vi "Autonomous Independent.vi"() -> ()   [LabVIEW 2016]
doc: "This VI is called when autonomous begins, and will automatically be terminated when autonomous ends. You can carry out timed or sensor driven robot movement independently without needing to return to the caller."
uses:
  <vilib>/Rock Robotics/WPI/Utilities/WPI_GetSetVariantRefNum.vi
  <vilib>/Rock Robotics/Network Tables/NT Read String.vi
  <vilib>/Rock Robotics/Network Tables/NT Write Numeric Array.vi
  <vilib>/Rock Robotics/WPI/RobotDrive/WPI_RobotDriveArcadeDrive_Standard(NoSaturation).vi
panel:
  out "Current Movement, for debugging":T1 {"Y Joystick Value" scale=1.0..-1.0; "X Joystick Value" scale=-1.0..1.0}
  in  "Array of robot movements":T2(array[cluster])=[{"X Joystick Value"=0.39393939393939403, "Y Joystick Value"=0.0, "Delay (sec)"=1.0, "Movement Name"="turn"}, {"X Joystick Value"=-0.3737373737373737, "Y Joystick Value"=0.0, "Delay (sec)"=1.0, "Movement Name"="turn back"}] {"Y Joystick Value" scale=1.0..-1.0; "X Joystick Value" scale=-1.0..1.0}
  # "Be sure to right-click and choose Data Operations>>Make Current Value default if you want to save the array values with the VI"
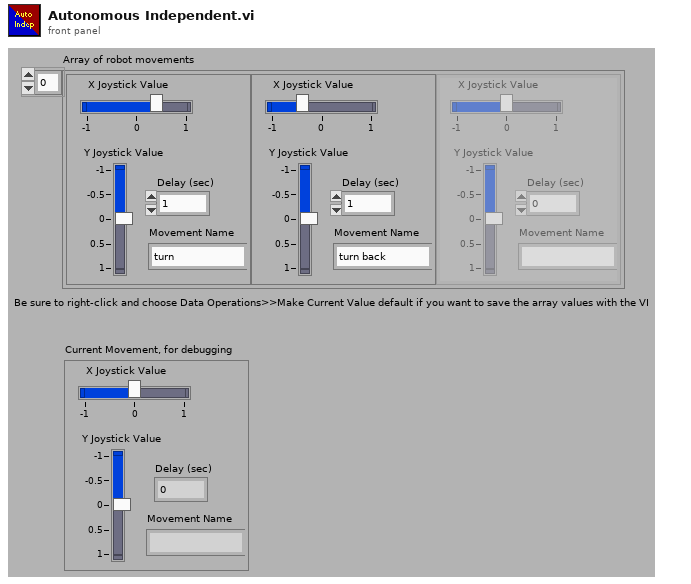
[diagram p1: front panel]
types:
  T1 = cluster{"X Joystick Value":dbl, "Y Joystick Value":dbl, "Delay (sec)":dbl, "Movement Name":string}
  T2 = cluster{"X Joystick Value":dbl, "Y Joystick Value":dbl, "Delay (sec)":dbl, "Movement Name":string}[]
  T3 = typedef "WPI_JoystickDevRef.ctl" = cluster{"Device":T4}
  T4 = typedef "WPI_JoystickDeviceEnum.ctl" = enum16{"USB 0", "USB 1", "USB 2", "USB 3", "USB 4", "USB 5"}
  T5 = typedef "WPI_RobotDriveDevRef.ctl" = cluster{"DevStatus":errorcluster, "Motors[]":T6[], "Square Inputs":bool, "Max Output":dbl}
  T6 = typedef "WPI_MotorControlDeviceRef.ctl" = cluster{"DeviceStatus":errorcluster, "Type":T7, "PWM":cluster{"PWM Channel":T8, "DeadBand":T9}, "CAN":cluster{"Device Number":u8, "SetOutput VI Ref":variant, "GetOutput VI Ref":variant, "Enable VI Ref":variant, "Disable VI Ref":variant, "Data":variant}, "Invert":bool}
  T7 = typedef "WPI_MotorControlType.ctl" = enum16{"PWM", "CAN"}
  T8 = typedef "FPGA_DIOPWMChannel.ctl" = enum8{"PWM 0", "PWM 1", "PWM 2", "PWM 3", "PWM 4", "PWM 5", "PWM 6", "PWM 7", "PWM 8", "PWM 9", "PWM MXP 0", "PWM MXP 1", "PWM MXP 2", "PWM MXP 3", "PWM MXP 4", "PWM MXP 5", "PWM MXP 6", "PWM MXP 7", "PWM MXP 8", "PWM MXP 9", "Invalid"}
  T9 = typedef "WPI_PWMDeadband.ctl" = cluster{"Name":string, "maxPositivePwm":i32, "minPositivePwm":i32, "centerPwm":i32, "maxNegativePwm":i32, "minNegativePwm":i32, "angularRange":u16}
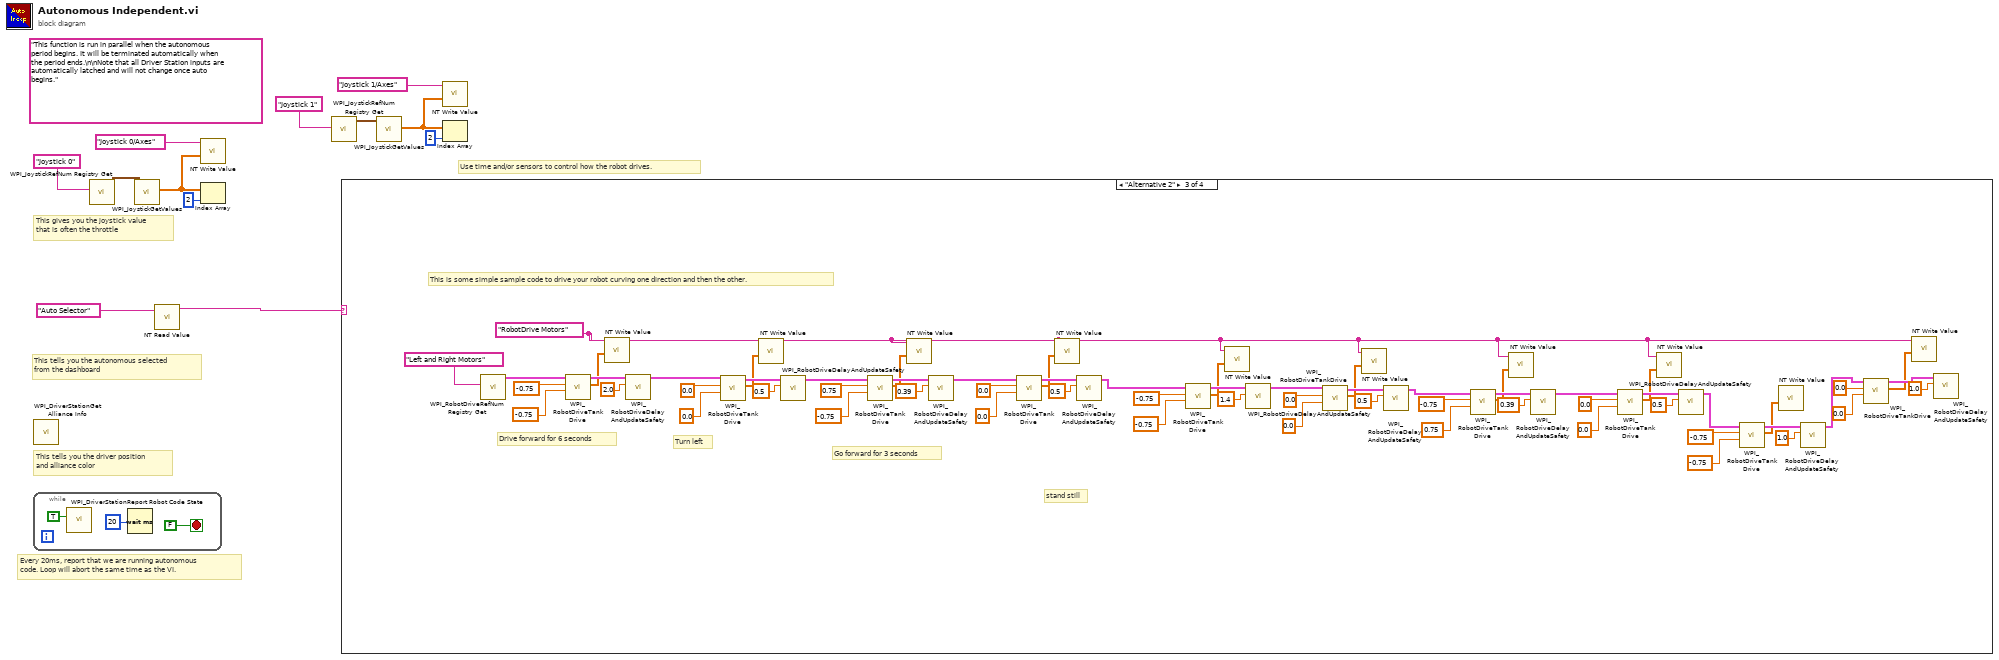
[diagram p0: block diagram]
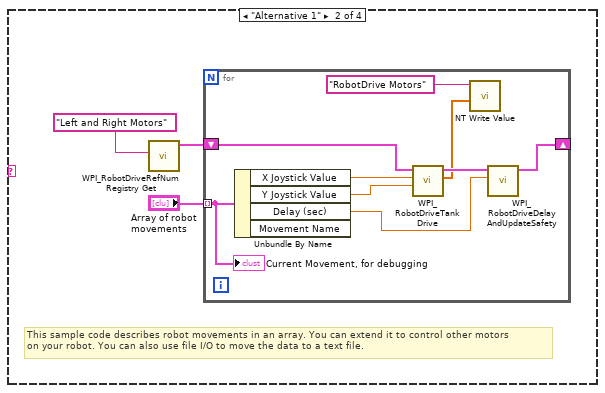
[diagram p3: hidden frame]
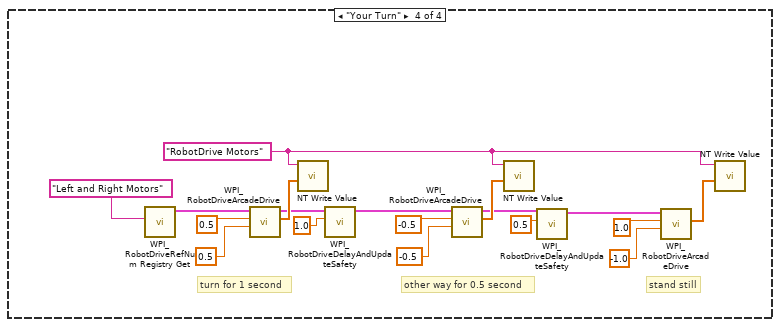
[diagram p4: hidden frame]
diagram:
  (unwired) "This function is run in parallel when the autonomous period begins. It will be terminated automatically when the period ends.\n\nNote that all Driver Station inputs are automatically latched and will not change once auto begins."
  # "This tells you the autonomous selected\nfrom the dashboard"
  # "Every 20ms, report that we are running autonomous\ncode. Loop will abort the same time as the VI."
  # "This gives you the joystick value\nthat is often the throttle"
  # "Use time and/or sensors to control how the robot drives."
  # "This tells you the driver position\nand alliance color"
  n1 = while {
    stop <- FALSE stop-if-true
    n2 = call <vilib>:"WPI_DriverStationReport Robot Code State.vi"("Autonomous"=TRUE) -> ()  [unwired: 10 in, 1 out]
    n3 = Wait (ms)(milliseconds to wait=u32 20) -> ()  [unwired: 1 out]
  }
  n4 = call <vilib>:"WPI_DriverStationGet Alliance Info.vi"() -> ()  [unwired: 12 out]
  n5 = call <vilib>:"WPI_JoystickRefNum Registry Get.vi"("refnum name"="Joystick 0") -> ("JoystickDevRef"=w11:T3)  [unwired: 1 in, 9 out]
  n6 = call <vilib>:"WPI_JoystickGetValues.vi"("JoystickDevRef"=w11) -> ("Axes"=w7:dbl[])  [unwired: 6 in, 4 out]
  n7 = call-poly <vilib>:"NT Read Value.vi"("Name"="Auto Selector") -> ("String"=w8:string)  [unwired: 9 in, 1 out]
  n8 = call-poly <vilib>:"NT Write Value.vi"("Numeric Array"=w7, "Name"="Joystick 0/Axes") -> ()  [unwired: 9 in, 1 out]
  n9 = Index Array(array=w7, index=2) -> ()  [unwired: 1 out]
  n10 = call <vilib>:"WPI_JoystickRefNum Registry Get.vi"("refnum name"="Joystick 1") -> ("JoystickDevRef"=w4:T3)  [unwired: 1 in, 9 out]
  n11 = case shown="\"Alternative 2\"" w8 {
    frame Default {
      # "You can put your main auto here, or you can right-click on the case and make any\nother frame be the default case."
      # "This is the frame that will execute if no selection is made, or if it is not recognized"
    }
    frame "Alternative 1" {
      # "This sample code describes robot movements in an array. You can extend it to control other motors\non your robot. You can also use file I/O to move the data to a text file."
      n12 = call <vilib>:"WPI_RobotDriveRefNum Registry Get.vi"("refnum name"="Left and Right Motors") -> ("RobotDriveDevRef"=w17:T5)  [unwired: 1 in, 9 out]
      n13 = for {
        shift-right: [w25] -> _
        shift-left: w17 -> [w26]
        tunnel: "Array of robot movements" -> [w21] mode=indexing
        n14 = Unbundle By Name(w21) -> ("X Joystick Value"=w24:dbl, "Y Joystick Value"=w23:dbl, "Delay (sec)"=w22:dbl)  [unwired: 1 out]
        n15 = call <vilib>:"WPI_RobotDriveTankDrive.vi"("Right axis value"=w23, "Left axis value"=w24, "RobotDriveDevRef"=w26) -> ("Motor Values"=w19:dbl[], "RobotDriveDevRef"=w27:T5)  [unwired: 6 in, 1 out]
        n16 = call-poly <vilib>:"NT Write Value.vi"("Numeric Array"=w19, "Name"="RobotDrive Motors") -> ()  [unwired: 9 in, 1 out]
        n17 = call <vilib>:"WPI_RobotDriveDelayAndUpdateSafety.vi"("Delay (s)"=w22, "RobotDriveDevRef"=w27) -> ("RobotDriveDevRef 2"=w25:T5)  [unwired: 8 in, 1 out]
        "Current Movement, for debugging" <- w21
      }
    }
    frame "Alternative 2" {
      w35 = "RobotDrive Motors" ("Name")
      # "Turn left"
      # "Go forward for 3 seconds"
      # "This is some simple sample code to drive your robot curving one direction and then the other."
      # "stand still"
      # "Drive forward for 6 seconds"
      n18 = call <vilib>:"WPI_RobotDriveRefNum Registry Get.vi"("refnum name"="Left and Right Motors") -> ("RobotDriveDevRef"=w89:T5)  [unwired: 1 in, 9 out]
      n19 = call <vilib>:"WPI_RobotDriveTankDrive.vi"("Right axis value"=-0.75 ("X axis value"), "Left axis value"=-0.75 ("X axis value"), "RobotDriveDevRef"=w89) -> ("Motor Values"=w83:dbl[], "RobotDriveDevRef"=w86:T5)  [unwired: 6 in, 1 out]
      n20 = call-poly <vilib>:"NT Write Value.vi"("Numeric Array"=w83, "Name"=w35) -> ()  [unwired: 9 in, 1 out]
      n21 = call <vilib>:"WPI_RobotDriveDelayAndUpdateSafety.vi"("Delay (s)"=2.0, "RobotDriveDevRef"=w86) -> ("RobotDriveDevRef 2"=w61:T5)  [unwired: 8 in, 1 out]
      n22 = call <vilib>:"WPI_RobotDriveTankDrive.vi"("Right axis value"=0.0 ("X axis value"), "Left axis value"=0.0 ("X axis value"), "RobotDriveDevRef"=w61) -> ("Motor Values"=w62:dbl[], "RobotDriveDevRef"=w65:T5)  [unwired: 6 in, 1 out]
      n23 = call-poly <vilib>:"NT Write Value.vi"("Numeric Array"=w62) -> ()  [unwired: 10 in, 1 out]
      n24 = call <vilib>:"WPI_RobotDriveDelayAndUpdateSafety.vi"("Delay (s)"=0.5, "RobotDriveDevRef"=w65) -> ("RobotDriveDevRef 2"=w60:T5)  [unwired: 8 in, 1 out]
      n25 = call <vilib>:"WPI_RobotDriveTankDrive.vi"("Right axis value"=-0.75 ("X axis value"), "Left axis value"=0.75 ("X axis value"), "RobotDriveDevRef"=w60) -> ("Motor Values"=w68:dbl[], "RobotDriveDevRef"=w71:T5)  [unwired: 6 in, 1 out]
      n26 = call-poly <vilib>:"NT Write Value.vi"("Numeric Array"=w68, "Name"=w35) -> ()  [unwired: 9 in, 1 out]
      n27 = call <vilib>:"WPI_RobotDriveDelayAndUpdateSafety.vi"("Delay (s)"=0.39, "RobotDriveDevRef"=w71) -> ("RobotDriveDevRef 2"=w67:T5)  [unwired: 8 in, 1 out]
      n28 = call <vilib>:"WPI_RobotDriveTankDrive.vi"("Right axis value"=0.0 ("X axis value"), "Left axis value"=0.0 ("X axis value"), "RobotDriveDevRef"=w67) -> ("Motor Values"=w73:dbl[], "RobotDriveDevRef"=w76:T5)  [unwired: 6 in, 1 out]
      n29 = call-poly <vilib>:"NT Write Value.vi"("Numeric Array"=w73, "Name"=w35) -> ()  [unwired: 9 in, 1 out]
      n30 = call <vilib>:"WPI_RobotDriveDelayAndUpdateSafety.vi"("Delay (s)"=0.5, "RobotDriveDevRef"=w76) -> ("RobotDriveDevRef 2"=w49:T5)  [unwired: 8 in, 1 out]
      n31 = call <vilib>:"WPI_RobotDriveTankDrive.vi"("Right axis value"=-0.75 ("X axis value"), "Left axis value"=-0.75 ("X axis value"), "RobotDriveDevRef"=w49) -> ("Motor Values"=w50:dbl[], "RobotDriveDevRef"=w53:T5)  [unwired: 6 in, 1 out]
      n32 = call-poly <vilib>:"NT Write Value.vi"("Numeric Array"=w50, "Name"=w35) -> ()  [unwired: 9 in, 1 out]
      n33 = call <vilib>:"WPI_RobotDriveDelayAndUpdateSafety.vi"("Delay (s)"=1.4, "RobotDriveDevRef"=w53) -> ("RobotDriveDevRef 2"=w48:T5)  [unwired: 8 in, 1 out]
      n34 = call <vilib>:"WPI_RobotDriveTankDrive.vi"("Right axis value"=0.0 ("X axis value"), "Left axis value"=0.0 ("X axis value"), "RobotDriveDevRef"=w48) -> ("Motor Values"=w55:dbl[], "RobotDriveDevRef"=w58:T5)  [unwired: 6 in, 1 out]
      n35 = call-poly <vilib>:"NT Write Value.vi"("Numeric Array"=w55, "Name"=w35) -> ()  [unwired: 9 in, 1 out]
      n36 = call <vilib>:"WPI_RobotDriveDelayAndUpdateSafety.vi"("Delay (s)"=0.5, "RobotDriveDevRef"=w58) -> ("RobotDriveDevRef 2"=w37:T5)  [unwired: 8 in, 1 out]
      n37 = call <vilib>:"WPI_RobotDriveTankDrive.vi"("Right axis value"=0.75 ("X axis value"), "Left axis value"=-0.75 ("X axis value"), "RobotDriveDevRef"=w37) -> ("Motor Values"=w38:dbl[], "RobotDriveDevRef"=w41:T5)  [unwired: 6 in, 1 out]
      n38 = call-poly <vilib>:"NT Write Value.vi"("Numeric Array"=w38, "Name"=w35) -> ()  [unwired: 9 in, 1 out]
      n39 = call <vilib>:"WPI_RobotDriveDelayAndUpdateSafety.vi"("Delay (s)"=0.39, "RobotDriveDevRef"=w41) -> ("RobotDriveDevRef 2"=w36:T5)  [unwired: 8 in, 1 out]
      n40 = call <vilib>:"WPI_RobotDriveTankDrive.vi"("Right axis value"=0.0 ("X axis value"), "Left axis value"=0.0 ("X axis value"), "RobotDriveDevRef"=w36) -> ("Motor Values"=w43:dbl[], "RobotDriveDevRef"=w46:T5)  [unwired: 6 in, 1 out]
      n41 = call-poly <vilib>:"NT Write Value.vi"("Numeric Array"=w43, "Name"=w35) -> ()  [unwired: 9 in, 1 out]
      n42 = call <vilib>:"WPI_RobotDriveDelayAndUpdateSafety.vi"("Delay (s)"=0.5, "RobotDriveDevRef"=w46) -> ("RobotDriveDevRef 2"=w29:T5)  [unwired: 8 in, 1 out]
      n43 = call <vilib>:"WPI_RobotDriveTankDrive.vi"("Right axis value"=-0.75 ("X axis value"), "Left axis value"=-0.75 ("X axis value"), "RobotDriveDevRef"=w29) -> ("Motor Values"=w30:dbl[], "RobotDriveDevRef"=w33:T5)  [unwired: 6 in, 1 out]
      n44 = call-poly <vilib>:"NT Write Value.vi"("Numeric Array"=w30) -> ()  [unwired: 10 in, 1 out]
      n45 = call <vilib>:"WPI_RobotDriveDelayAndUpdateSafety.vi"("Delay (s)"=1.0, "RobotDriveDevRef"=w33) -> ("RobotDriveDevRef 2"=w28:T5)  [unwired: 8 in, 1 out]
      n46 = call <vilib>:"WPI_RobotDriveTankDrive.vi"("Right axis value"=0.0 ("X axis value"), "Left axis value"=0.0 ("X axis value"), "RobotDriveDevRef"=w28) -> ("Motor Values"=w78:dbl[], "RobotDriveDevRef"=w81:T5)  [unwired: 6 in, 1 out]
      n47 = call-poly <vilib>:"NT Write Value.vi"("Numeric Array"=w78, "Name"=w35) -> ()  [unwired: 9 in, 1 out]
      n48 = call <vilib>:"WPI_RobotDriveDelayAndUpdateSafety.vi"("Delay (s)"=1.0, "RobotDriveDevRef"=w81) -> ()  [unwired: 8 in, 2 out]
    }
    frame "Your Turn" {
      w106 = "RobotDrive Motors" ("Name")
      # "stand still"
      # "other way for 0.5 second"
      # "turn for 1 second"
      n49 = call <vilib>:"WPI_RobotDriveRefNum Registry Get.vi"("refnum name"="Left and Right Motors") -> ("RobotDriveDevRef"=w90:T5)  [unwired: 1 in, 9 out]
      n50 = call-poly <vilib>:"WPI_RobotDriveArcadeDrive.vi"("Y axis value"=0.5 ("X axis value"), "X axis value"=0.5, "RobotDriveDevRef"=w90) -> ("Motor Values"=w107:dbl[], "RobotDriveDevRef"=w97:T5)  [unwired: 1 in, 6 out]
      n51 = call-poly <vilib>:"NT Write Value.vi"("Numeric Array"=w107, "Name"=w106) -> ()  [unwired: 9 in, 1 out]
      n52 = call <vilib>:"WPI_RobotDriveDelayAndUpdateSafety.vi"("Delay (s)"=1.0, "RobotDriveDevRef"=w97) -> ("RobotDriveDevRef 2"=w96:T5)  [unwired: 8 in, 1 out]
      n53 = call-poly <vilib>:"WPI_RobotDriveArcadeDrive.vi"("Y axis value"=-0.5 ("X axis value"), "X axis value"=-0.5, "RobotDriveDevRef"=w96) -> ("Motor Values"=w105:dbl[], "RobotDriveDevRef"=w95:T5)  [unwired: 1 in, 6 out]
      n54 = call-poly <vilib>:"NT Write Value.vi"("Numeric Array"=w105, "Name"=w106) -> ()  [unwired: 9 in, 1 out]
      n55 = call <vilib>:"WPI_RobotDriveDelayAndUpdateSafety.vi"("Delay (s)"=0.5, "RobotDriveDevRef"=w95) -> ("RobotDriveDevRef 2"=w94:T5)  [unwired: 8 in, 1 out]
      n56 = call-poly <vilib>:"WPI_RobotDriveArcadeDrive.vi"("Y axis value"=-1.0 ("X axis value"), "X axis value"=1.0, "RobotDriveDevRef"=w94) -> ("Motor Values"=w104:dbl[])  [unwired: 1 in, 7 out]
      n57 = call-poly <vilib>:"NT Write Value.vi"("Numeric Array"=w104, "Name"=w106) -> ()  [unwired: 9 in, 1 out]
    }
  }
  n58 = call <vilib>:"WPI_JoystickGetValues.vi"("JoystickDevRef"=w4) -> ("Axes"=w2:dbl[])  [unwired: 6 in, 4 out]
  n59 = call-poly <vilib>:"NT Write Value.vi"("Numeric Array"=w2, "Name"="Joystick 1/Axes") -> ()  [unwired: 9 in, 1 out]
  n60 = Index Array(array=w2, index=2) -> ()  [unwired: 1 out]
